vi "Parameters_Build_VelocityMove.vi"(9 "Acceleration Jerk":dbl=1000.0, 10 "Acceleration":dbl=10000.0, 11 "Velocity":dbl=1000.0) -> (3 "Parameters":dbl[](array[numeric]))   [LabVIEW 2017, in "WordManipulationLibrary.lvlib"]
uses:
  WordManipulationLibrary.lvlib
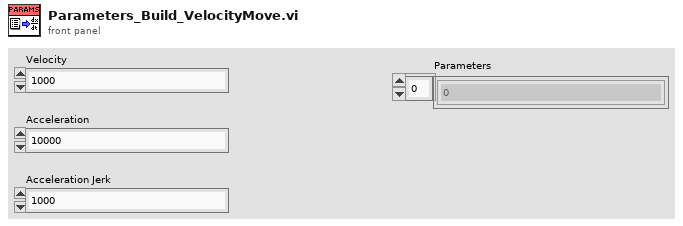
[diagram p1: front panel]
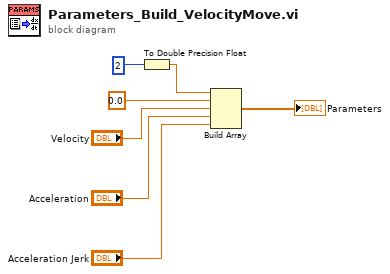
[diagram p0: block diagram]
diagram:
  n1 = To Double Precision Float(number=i16 2 ("element")) -> (double precision float=w5:dbl)
  n2 = Build Array(w5, 0.0 ("element"), "Velocity", "Acceleration", "Acceleration Jerk") -> (→"Parameters":dbl[])
